vi "ShowWindow.vi"(8 "error in (no error)":errorcluster, 10 "nCmdShow\n(SW_SHOWNORMAL)":T1(ring)=enum."SW_SHOWNORMAL", 11 "hWnd (NULL)":T2) -> (0 "error out":errorcluster, 2 "Previously Visible?":bool, 3 "dup hWnd":T2)   [LabVIEW 2011]
doc: "ShowWindow\nThe ShowWindow function sets the specified window's show state. \n\nBOOL ShowWindow(\n HWND hWnd, // handle to window\n int nCmdShow // show state of window\n);\n \nParameters\nhWnd \nHandle to the window. \nnCmdShow \nSpecifies how the window is to be shown. This parameter is ignored the first time an application calls ShowWindow, if the program that launched the application provides aSTARTUPINFO structure. Otherwise, the first time ShowWindow is called, the value should be the value obtained by the WinMain function in its nCmdShow parameter. In subsequent calls, this parameter can be one of the following values: Value Meaning \nSW_FORCEMINIMIZE Windows NT 5.0 and later: Minimizes a window, even if the thread that owns the window is hung. This flag should only be used when minimizing windows from a different thread. \nSW_HIDE Hides the window and activates another window. \nSW_MAXIMIZE Maximizes the specified window. \nSW_MINIMIZE Minimizes the specified window and activates the next top-level window in the Z order. \nSW_RESTORE Activates and displays the window. If the window is minimized or maximized, the system restores it to its original size and position. An application should specify this flag when restoring a minimized window. \nSW_SHOW Activates the window and displays it in its current size and position. \nSW_SHOWDEFAULT Sets the show state based on the SW_ flag specified in theSTARTUPINFO structure passed to theCreateProcess function by the program that started the application. \nSW_SHOWMAXIMIZED Activates the window and displays it as a maximized window. \nSW_SHOWMINIMIZED Activates the window and displays it as a minimized window. \nSW_SHOWMINNOACTIVE Displays the window as a minimized window. The active window remains active. \nSW_SHOWNA Displays the window in its current state. The active window remains active. \nSW_SHOWNOACTIVATE Displays a window in its most recent size and position. The active window remains active. \nSW_SHOWNORMAL Activates and displays a window. If the window is minimized or maximized, the system restores it to its original size and position. An application should specify this flag when displaying the window for the first time. \n\n\nReturn Values\nIf the window was previously visible, the return value is nonzero. \n\nIf the window was previously hidden, the return value is zero. \n\nRemarks\nThe first time an application calls ShowWindow, it should use the WinMain function's nCmdShow parameter as its nCmdShow parameter. Subsequent calls to ShowWindow must use one of the values in the given list, instead of the one specified by the WinMain function's nCmdShow parameter. \n\nAs noted in the discussion of the nCmdShow parameter, the nCmdShow value is ignored in the first call to ShowWindow if the program that launched the application specifies startup information in theSTARTUPINFO structure. In this case, ShowWindow uses the information specified in the STARTUPINFO structure to show the window. On subsequent calls, the application must call ShowWindow with nCmdShow set to SW_SHOWDEFAULT to use the startup information provided by the program that launched the application. This behavior is designed for the following situations: \n\nApplications create their main window by calling CreateWindow with the WS_VISIBLE flag set. \nApplications create their main window by calling CreateWindow with the WS_VISIBLE"
uses:
  hWnd.ctl
  user32.dll
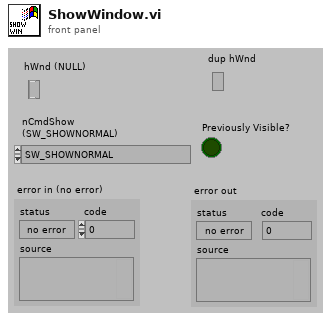
[diagram p1: front panel]
types:
  T1 = enum32{"SW_SHOWDEFAULT", "SW_FORCEMINIMIZE", "SW_HIDE", "SW_MAXIMIZE", "SW_RESTORE", "SW_SHOW", "SW_SHOWMAXIMIZED", "SW_SHOWMINIMIZED", "SW_SHOWMINNOACTIVE", "SW_SHOWNA", "SW_SHOWNOACTIVATE", "SW_SHOWNORMAL"}
  T2 = typedef "hWnd.ctl" = refnum<k1>
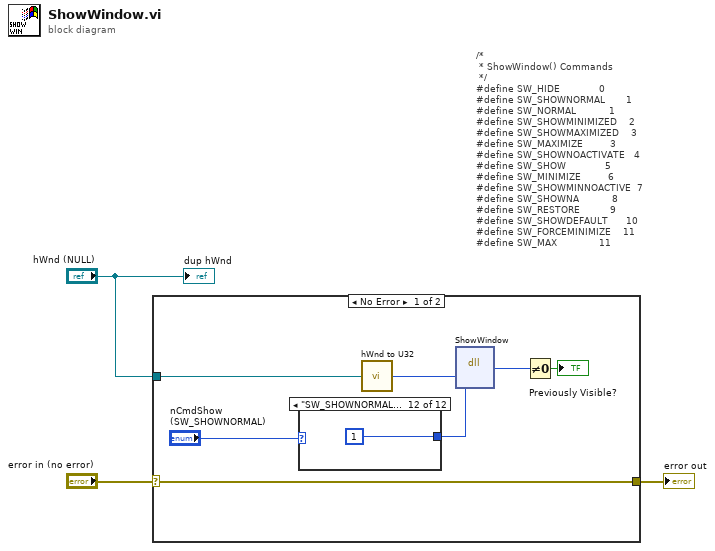
[diagram p0: block diagram]
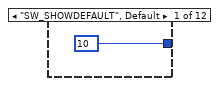
[diagram p2: hidden frame]
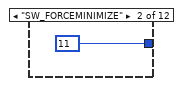
[diagram p3: hidden frame]
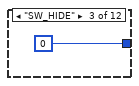
[diagram p4: hidden frame]
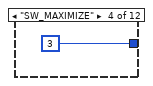
[diagram p5: hidden frame]
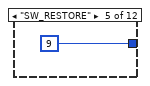
[diagram p6: hidden frame]
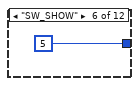
[diagram p7: hidden frame]
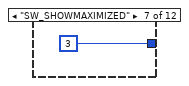
[diagram p8: hidden frame]
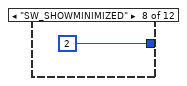
[diagram p9: hidden frame]
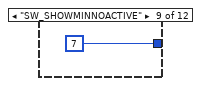
[diagram p10: hidden frame]
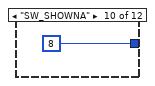
[diagram p11: hidden frame]
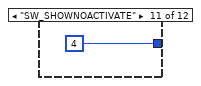
[diagram p12: hidden frame]
diagram:
  # "/*\n * ShowWindow() Commands\n */\n#define SW_HIDE             0\n#define SW_SHOWNORMAL       1\n#define SW_NORMAL           1\n#define SW_SHOWMINIMIZED    2\n#define SW_SHOWMAXIMIZED    3\n#define SW_MAXIMIZE         3\n#define SW_SHOWNOACTIVATE   4\n#define SW_SHOW             5\n#define SW_MINIMIZE         6\n#define SW_SHOWMINNOACTIVE  7\n#define SW_SHOWNA           8\n#define SW_RESTORE          9\n#define SW_SHOWDEFAULT      10\n#define SW_FORCEMINIMIZE    11\n#define SW_MAX              11"
  n1 = case shown="No Error" "error in (no error)" {
    selector: "error in (no error)" -> [w6 w23]
    tunnel: [w6 w23] -> w2
    tunnel: "hWnd (NULL)" -> [w7 _]
    frame No Error {
      n2 = case shown="\"SW_SHOWNORMAL\"" "nCmdShow\n(SW_SHOWNORMAL)" {
        tunnel: [10 11 0 3 9 5 3 2 7 8 4 1] -> w9
        frame "SW_SHOWDEFAULT", Default {
        }
        frame "SW_FORCEMINIMIZE" {
        }
        frame "SW_HIDE" {
        }
        frame "SW_MAXIMIZE" {
        }
        frame "SW_RESTORE" {
        }
        frame "SW_SHOW" {
        }
        frame "SW_SHOWMAXIMIZED" {
        }
        frame "SW_SHOWMINIMIZED" {
        }
        frame "SW_SHOWMINNOACTIVE" {
        }
        frame "SW_SHOWNA" {
        }
        frame "SW_SHOWNOACTIVATE" {
        }
        frame "SW_SHOWNORMAL" {
        }
      }
      n3 = call "hWnd to U32.vi"("hWnd"=w7) -> ("hWnd"=w8:u32)  [unwired: 4 out]
      n4 = dll-call lib="user32.dll" fn="ShowWindow"("hWnd"=w8, "nCmdShow"=w9) -> ("return type"=w5:i32)  [unwired: 5 in, 2 out]
      n5 = Not Equal To 0?(x=w5) -> (x != 0?=→"Previously Visible?":bool)
    }
    frame Error {
    }
  }
  "error out" <- w2
  "dup hWnd" <- "hWnd (NULL)"
